vi "初始化表格颜色.vi"(8 "错误输入（无错误）":errorcluster, 9 "选中颜色盒":u32(colorbox)=12439011, 10 "行列范围":cluster{"起始行列":T1, "结束行列":T1}, 11 "引用输入":refnum<vi>) -> (0 "错误输出":errorcluster, 3 "引用输出":refnum<vi>)   [LabVIEW 2014, in "表格.lvlib" / "表格上色.lvlib"]
uses:
  <vilib>/Utility/miscctls.llb/LVRowAndColumnTypeDef.ctl
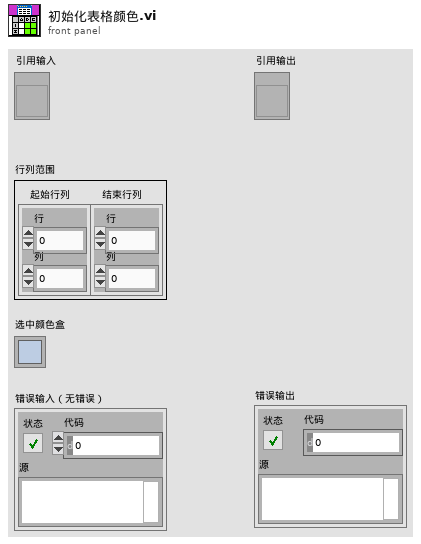
[diagram p1: front panel]
types:
  T1 = typedef "LVRowAndColumnTypeDef.ctl" = cluster{"Row":i32, "Column":i32}
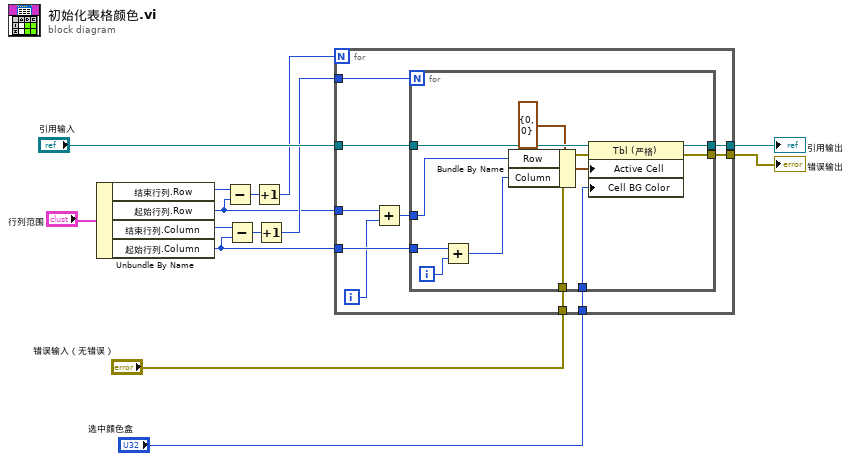
[diagram p0: block diagram]
diagram:
  n1 = Unbundle By Name("行列范围") -> ("结束行列.Row"=w8:i32, "起始行列.Row"=w2:i32, "结束行列.Column"=w5:i32, "起始行列.Column"=w1:i32)
  n2 = Subtract(x=w8, y=w2) -> (x-y=w6:i32)
  n3 = Subtract(x=w5, y=w1) -> (x-y=w7:i32)
  n4 = Increment(x=w6) -> (x+1=w4:i32)
  n5 = Increment(x=w7) -> (x+1=w3:i32)
  n6 = for {
    N: w4 -> [_]
    tunnel: "错误输入（无错误）" -> [w24]
    tunnel: [w23] -> w13
    tunnel: [w22] -> w12
    tunnel: "引用输入" -> [w21]
    tunnel: "选中颜色盒" -> [w20]
    tunnel: w3 -> [w19]
    tunnel: w2 -> [w17]
    tunnel: w1 -> [w18]
    i -> [w16]
    n7 = Add(x=w17, y=w16) -> (x+y=w15:i32)
    n8 = for {
      N: w19 -> [_]
      tunnel: w24 -> [w35]
      tunnel: [w34] -> w23
      tunnel: [w33] -> w22
      tunnel: w21 -> [w32]
      tunnel: w20 -> [w31]
      tunnel: w18 -> [w27]
      tunnel: w15 -> [w25]
      i -> [w28]
      n9 = Add(x=w27, y=w28) -> (x+y=w26:i32)
      n10 = Bundle By Name(cluster=T1 {"Row"=0, "Column"=0} ("活动单元格:活动单元格"), "Row"=w25, "Column"=w26) -> (w30:T1)
      n11 = property on="属性节点" class="Tbl (严格)"(reference=w32, error in=w35, "Active Cell"=w30, "Cell BG Color"=w31) -> (reference out=w33:refnum<vi>, error out=w34:errorcluster)
    }
  }
  "错误输出" <- w13
  "引用输出" <- w12
